vi "image_data_scaler.vi"(1 "Scale":dbl=1.0, 2 "Data In":cluster{"X":dbl, "Y":dbl}[][](array[cluster])) -> (0 "Data Out":cluster{"X":dbl, "Y":dbl}[][](array[cluster]))   [LabVIEW 2017]
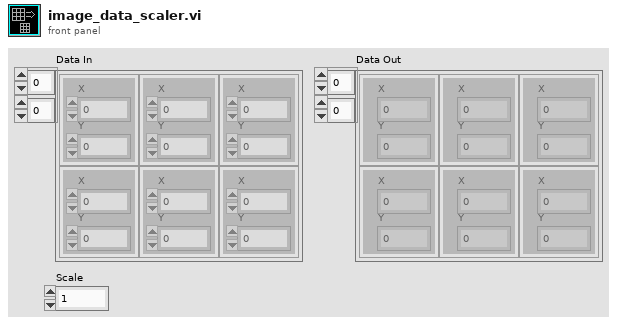
[diagram p1: front panel]
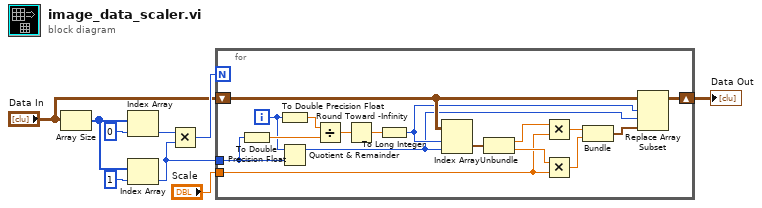
[diagram p0: block diagram]
diagram:
  n1 = Array Size(array="Data In") -> (size(s)=w8:i32[])
  n2 = Index Array(array=w8, index=0) -> (element=w5:i32)
  n3 = Index Array(array=w8, index=1) -> (element=w4:i32)
  n4 = Multiply(x=w5, y=w4) -> (x*y=w9:i32)
  n5 = for {
    N: w9 -> [_]
    shift-right: [w19] -> w2
    shift-left: "Data In" -> [w20]
    tunnel: w4 -> [w15]
    tunnel: "Scale" -> [w10]
    i -> [w22]
    n6 = To Double Precision Float(number=w15) -> (double precision float=w23:dbl)
    n7 = To Double Precision Float(number=w22) -> (double precision float=w24:dbl)
    n8 = Quotient & Remainder(x=w22, y=w15) -> (x-y*floor(x/y)=w16:i32)  [unwired: 1 out]
    n9 = Divide(x=w24, y=w23) -> (x/y=w26:dbl)
    n10 = Round Toward -Infinity(1:w26) -> (0:w25:dbl)
    n11 = To Long Integer(number=w25) -> (32bit integer=w17:i32)
    n12 = Index Array(array=w20, index (row)=w17, index (col)=w16) -> (element=w21:cluster{"X":dbl, "Y":dbl})
    n13 = Unbundle(w21) -> ("X"=w11:dbl, "Y"=w12:dbl)
    n14 = Multiply(x=w11, y=w10) -> (x*y=w14:dbl)
    n15 = Multiply(x=w12, y=w10) -> (x*y=w13:dbl)
    n16 = Bundle(w14, w13) -> (w18:cluster{dbl, dbl})  [unwired: 1 in]
    n17 = Replace Array Subset(array=w20, new element=w18, index (row)=w17, index (col)=w16) -> (w19:cluster{"X":dbl, "Y":dbl}[][])
  }
  "Data Out" <- w2
